vi "LaunchErrorLogger.vi"(8 "error in (no error)":errorcluster, 11 "TCP_Client in":refnum<class "TCP_Client.lvclass">) -> (0 "error out":errorcluster, 3 "TCP_Client out":refnum<class "TCP_Client.lvclass">)   [LabVIEW 2023, in "TCP_Client.lvlib" / "TCP_Client.lvclass"]
uses:
  TCP_Client.lvclass
  SimpleErrorLogger/SimpleErrorLogger/SimpleErrorLogger.lvclass
  TCP_Client.lvclass/TCP_Client.ctl
  SimpleErrorLogger/SimpleErrorLogger Messages/Write folder Msg/Write folder Msg.lvclass/Write folder Msg.ctl
  <vilib>/ActorFramework/Message Enqueuer/Message Enqueuer.lvclass/Message Enqueuer.ctl
  SimpleErrorLogger/SimpleErrorLogger Messages/Write filename Msg/Write filename Msg.lvclass/Write filename Msg.ctl
  <vilib>/ActorFramework/Message Enqueuer/Enqueue.vi
  SimpleErrorLogger/SimpleErrorLogger Messages/Write folder Msg/Write folder Msg.lvclass
  SimpleErrorLogger/SimpleErrorLogger Messages/Write filename Msg/Write filename Msg.lvclass
  SimpleErrorLogger/SimpleErrorLogger Messages/Open Msg/Open Msg.lvclass
  <vilib>/ActorFramework/Message Priority Queue/Priority Enqueue.vi
  <vilib>/ActorFramework/Actor/Actor.lvclass
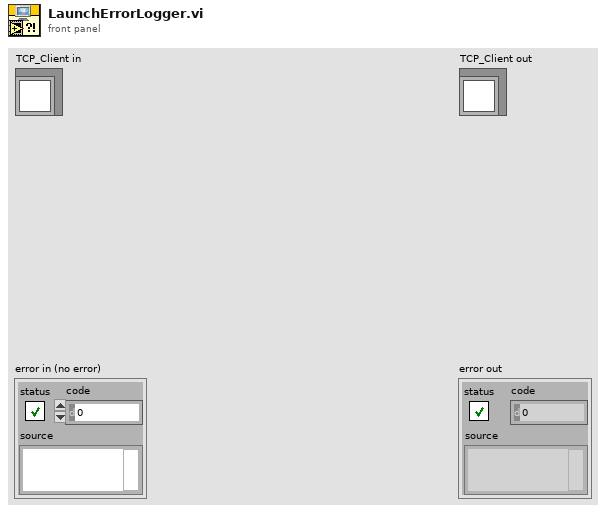
[diagram p1: front panel]
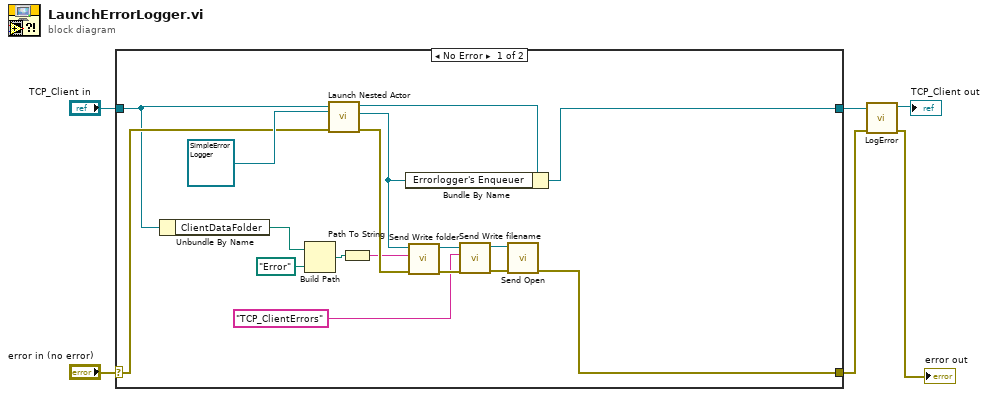
[diagram p0: block diagram]
diagram:
  n1 = case shown="No Error" "error in (no error)" {
    selector: "error in (no error)" -> [w22 w25]
    tunnel: [w12 w25] -> w2
    tunnel: [w20 w24] -> w4
    tunnel: "TCP_Client in" -> [w11 w24]
    frame No Error {
      n2 = Unbundle By Name(w11) -> ("ClientDataFolder"=w10:path)
      n3 = Build Path(base path=w10, name or relative path=path "Error") -> (appended path=w8:path)
      n4 = call <vilib>:"Launch Nested Actor.vi"("error in (no error)"=w22, "Nested Actor"=refnum<class "SimpleErrorLogger.lvclass"> refnum ("SimpleErrorLogger.lvlib:SimpleErrorLogger.lvclass"), "Caller Actor in"=w11) -> ("error out"=w13:errorcluster, "Nested Actor's Enqueuer"=w19:refnum<class "Message Enqueuer.lvclass">, "Caller Actor out"=w21:refnum<class "TCP_Client.lvclass">)  [unwired: 6 in]
      n5 = Path To String(path=w8) -> (string=w7:string)
      n6 = Bundle By Name(cluster=w21, "Errorlogger's Enqueuer"=w19) -> (w20:refnum<class "TCP_Client.lvclass">)
      n7 = call "Send Write folder.vi"("error in (no error)"=w13, "folder"=w7, "Message Enqueuer"=w19) -> ("error out"=w17:errorcluster, "Message Enqueuer out"=w18:refnum<class "Message Enqueuer.lvclass">)  [unwired: 7 in]
      n8 = call "Send Write filename.vi"("error in (no error)"=w17, "filename"="TCP_ClientErrors", "Message Enqueuer"=w18) -> ("error out"=w14:errorcluster, "Message Enqueuer out"=w15:refnum<class "Message Enqueuer.lvclass">)  [unwired: 7 in]
      n9 = call "Send Open.vi"("error in (no error)"=w14, "Message Enqueuer"=w15) -> ("error out"=w12:errorcluster)  [unwired: 8 in, 1 out]
    }
    frame Error {
    }
  }
  n10 = call "LogError.vi"("error in (no error)"=w2, "TCP_Client in"=w4) -> ("error out"=→"error out":errorcluster, "TCP_Client out"=→"TCP_Client out":refnum<class "TCP_Client.lvclass">)  [unwired: 8 in]
